vi "新记录通知.vi"() -> ()   [LabVIEW 2017]
uses:
  <vilib>/Utility/miscctls.llb/LVRowAndColumnTypeDef.ctl
  <vilib>/Utility/miscctls.llb/LVRowAndColumnUnsignedTypeDef.ctl
  <vilib>/Utility/inputDevices.llb/mouseAcquire.vi
panel:
  in  "列表菜单":enum16{"预览", "忽略此条", "删除缓存文件", "复制到剪贴板"}(ring)
  out "点到行列-实时列表":T1 caption="单元格位置"
  in  "device ID":refnum<k1> caption="设备ID"
  in  "新记录":cluster{"新记录列表行":string[], "对应缓存文件":string}[](array[cluster])
  in  "报警记录列表":i32[](listbox)
  in  "忽略全部":bool
  in  "预览全部":bool
  # "* 双击单元格打开预览\n  右键菜单中查看更多选项，管理界面中查看更多记录"
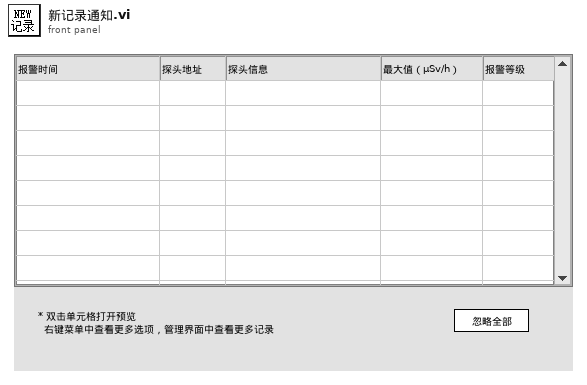
[diagram p1: front panel]
types:
  T1 = typedef "LVRowAndColumnTypeDef.ctl" = cluster{"Row":i32, "Column":i32}
  T2 = typedef "LVRowAndColumnUnsignedTypeDef.ctl" = cluster{"Row":u32, "Column":u32}
  T3 = enum32{"Invalid", "Standard", "Closed", "Hidden", "Minimized", "Maximized"}
  T4 = typedef "eventvkey.ctl" = enum16{"ASCII", "Enter", "Return", "Shift", "Ctrl", "Alt", "Cmd", "Opt", "Caps", "NumLock", "Clear", "Break", "Up", "Down", "Left", "Right", "Insert", "Delete", "Home", "End", "PageUp", "PageDown", "Escape", "Help", "Pause", "ScrollLock", "F1", "F2", "F3", "F4", "F5", "F6", "F7", "F8", "F9", "F10", "F11", "F12", "F13", "F14", "F15", "F16", "F17", "F18", "F19", "F20", "F21", "F22", "F23", "F24", "Play", "VolumeUp", "VolumeDown", "Mute", "Two Byte Char"}
  T5 = typedef "LVPoint32TypeDef.ctl" = cluster{"Horizontal":i32, "Vertical":i32}
  T6 = cluster{"button 1":bool, "button 2":bool, "button 3":bool, "button 4":bool}
  T7 = cluster{"Shift":bool, "Ctrl":bool, "Alt":bool, "Cmd":bool, "Opt":bool}
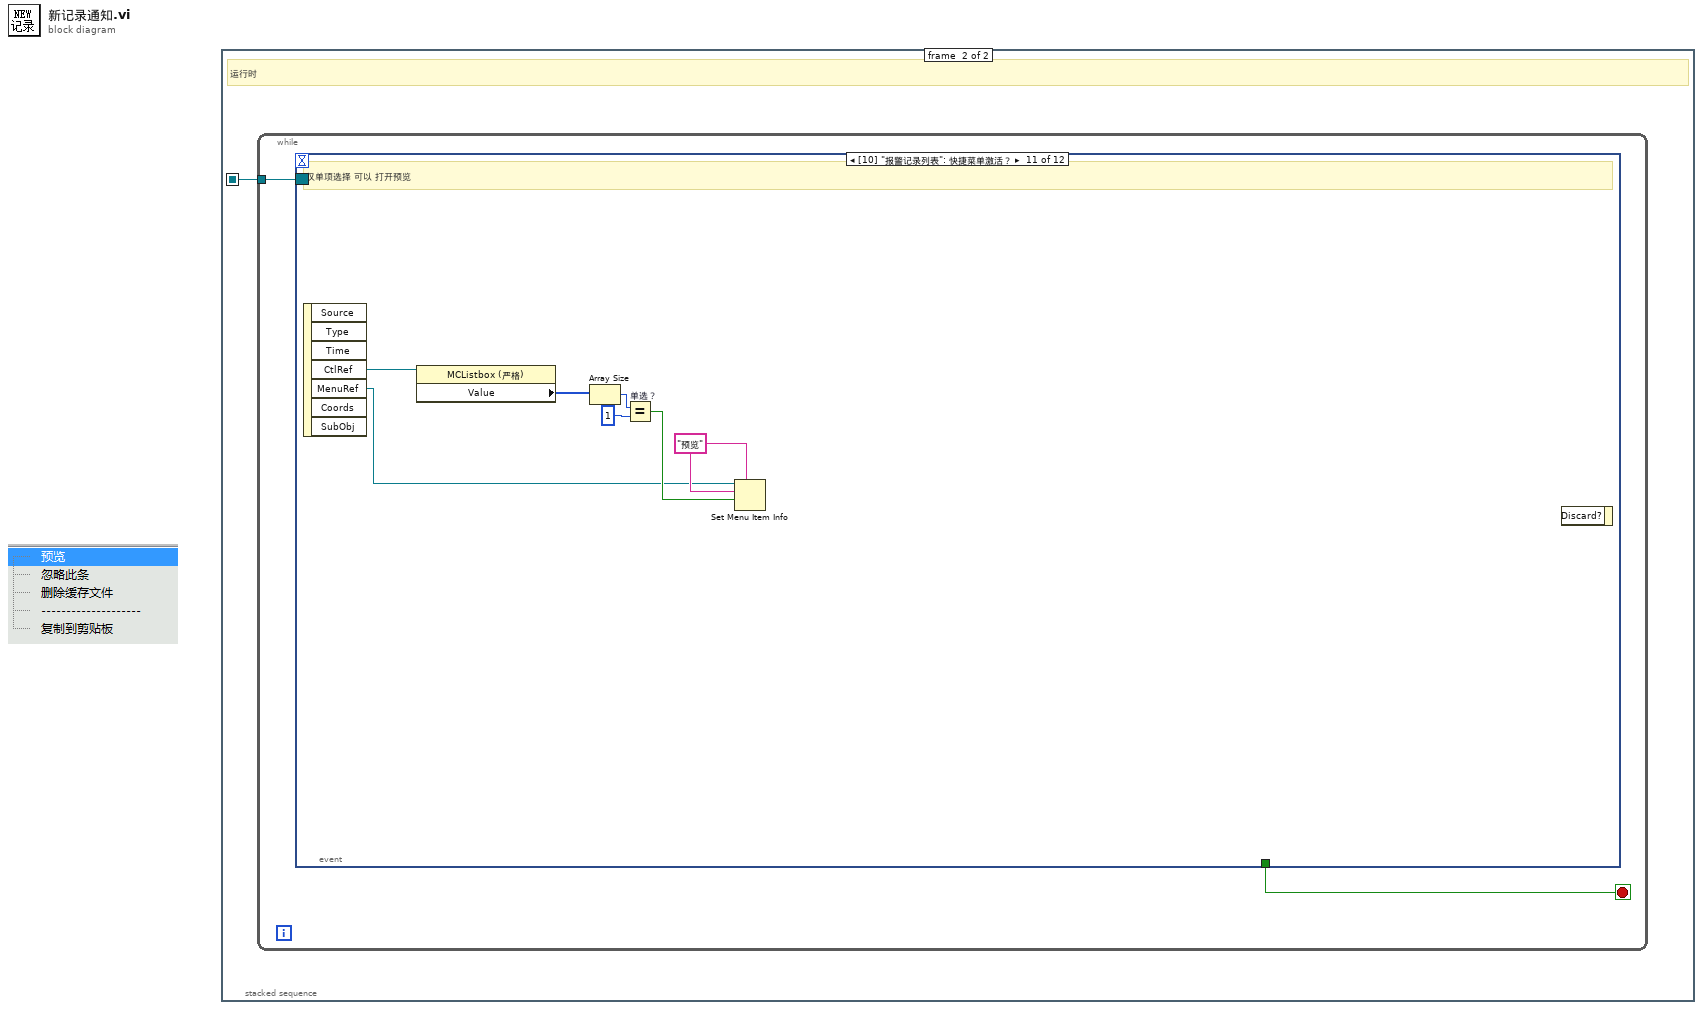
[diagram p0: block diagram]
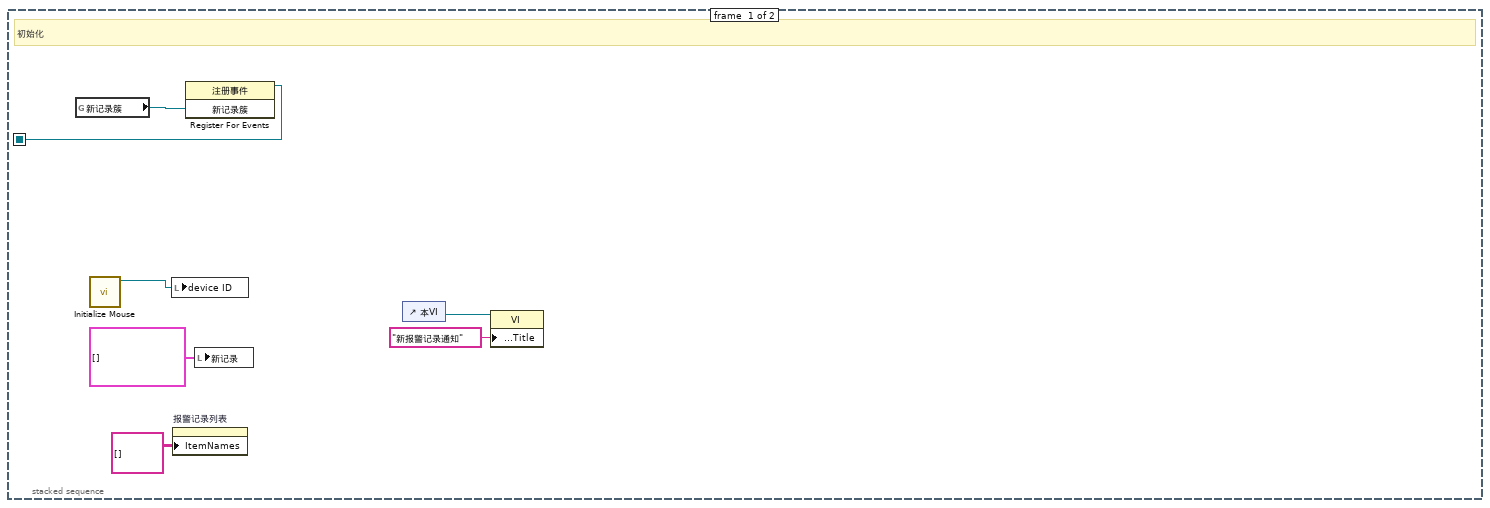
[diagram p2: hidden frame]
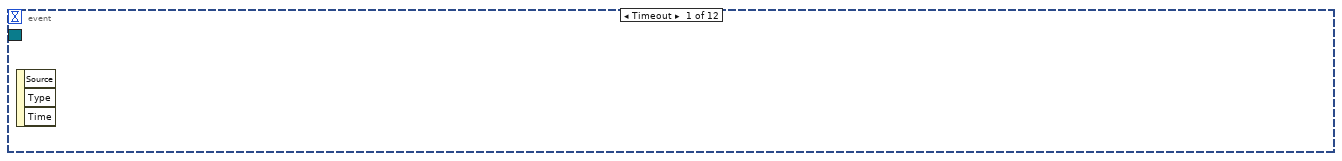
[diagram p3: hidden frame]
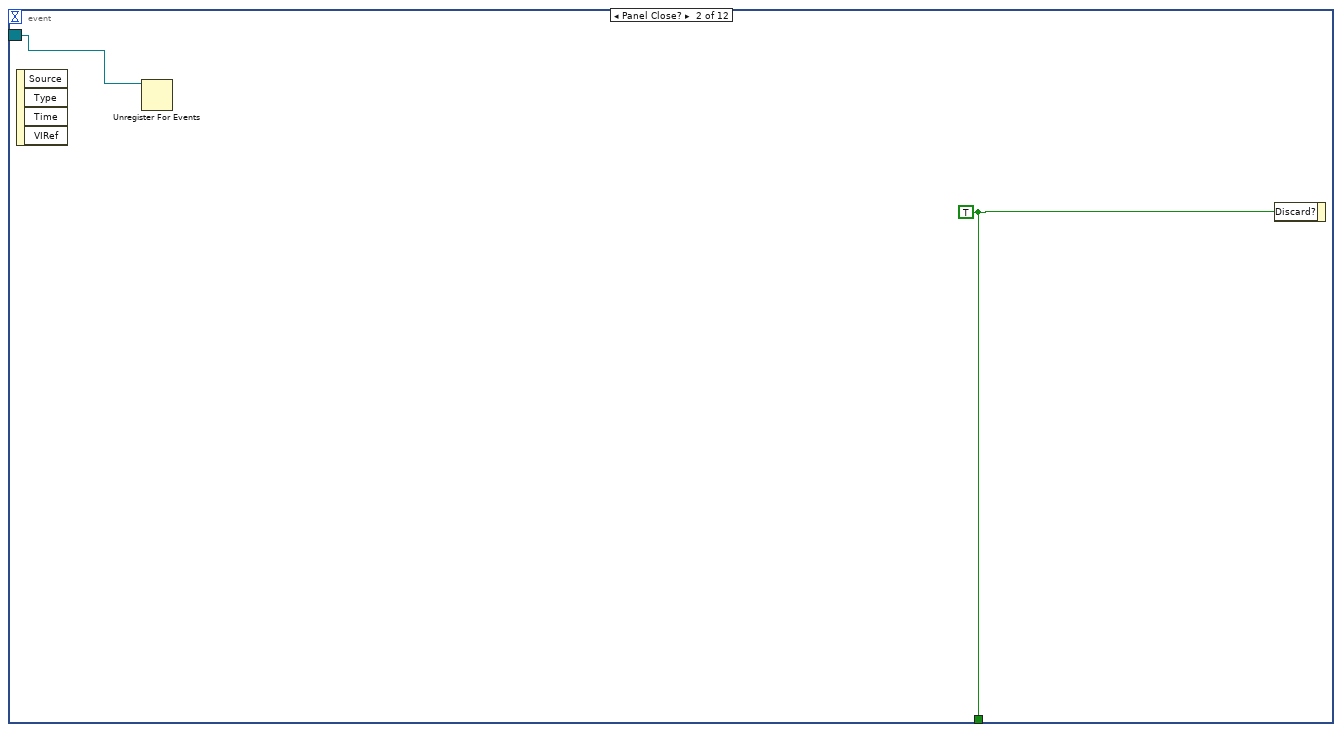
[diagram p4: hidden frame]
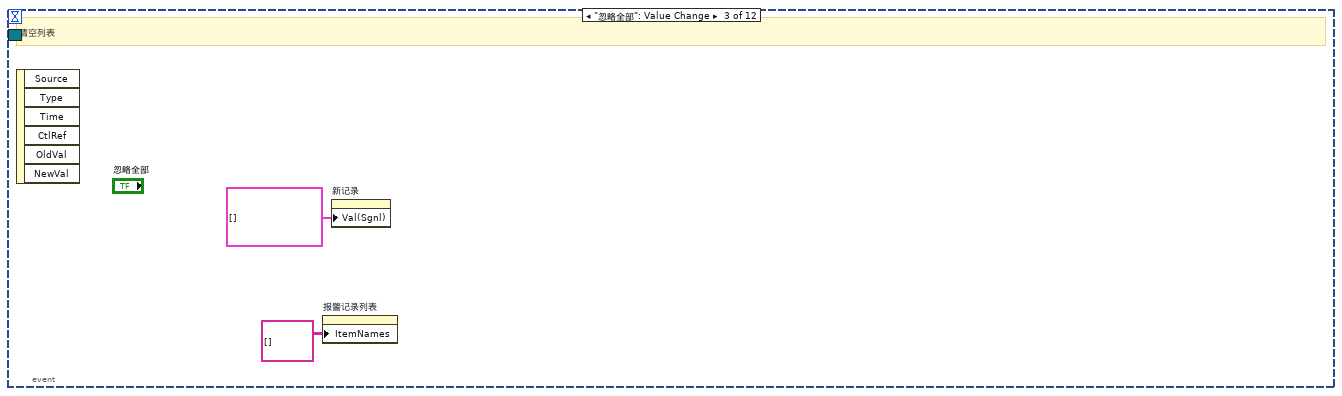
[diagram p5: hidden frame]
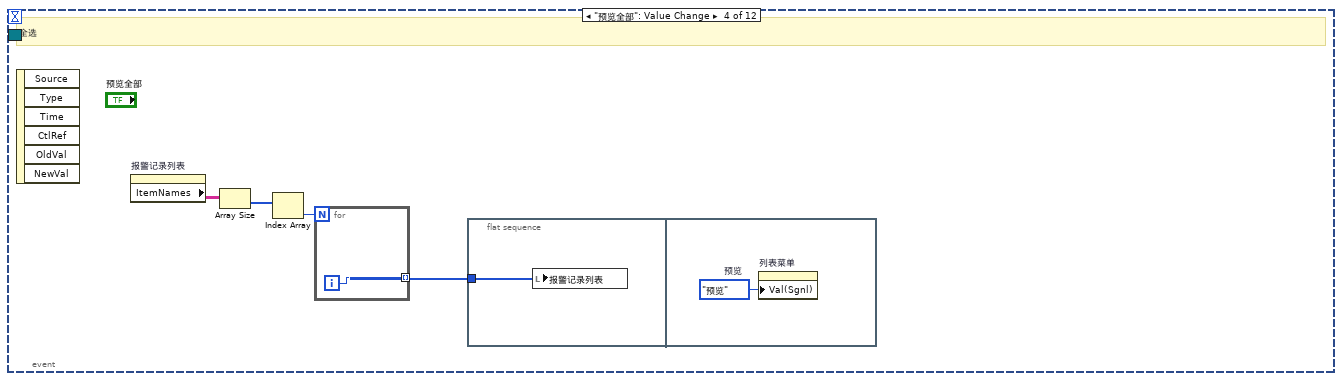
[diagram p6: hidden frame]
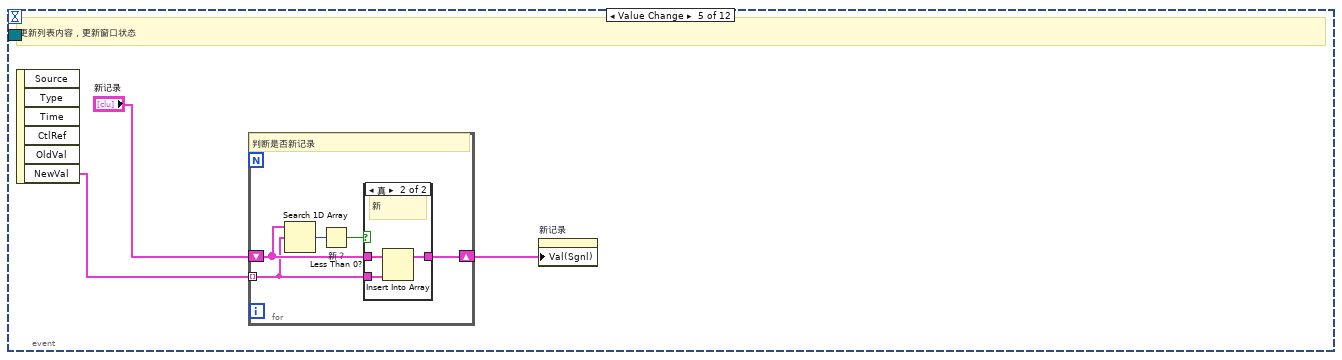
[diagram p7: hidden frame]
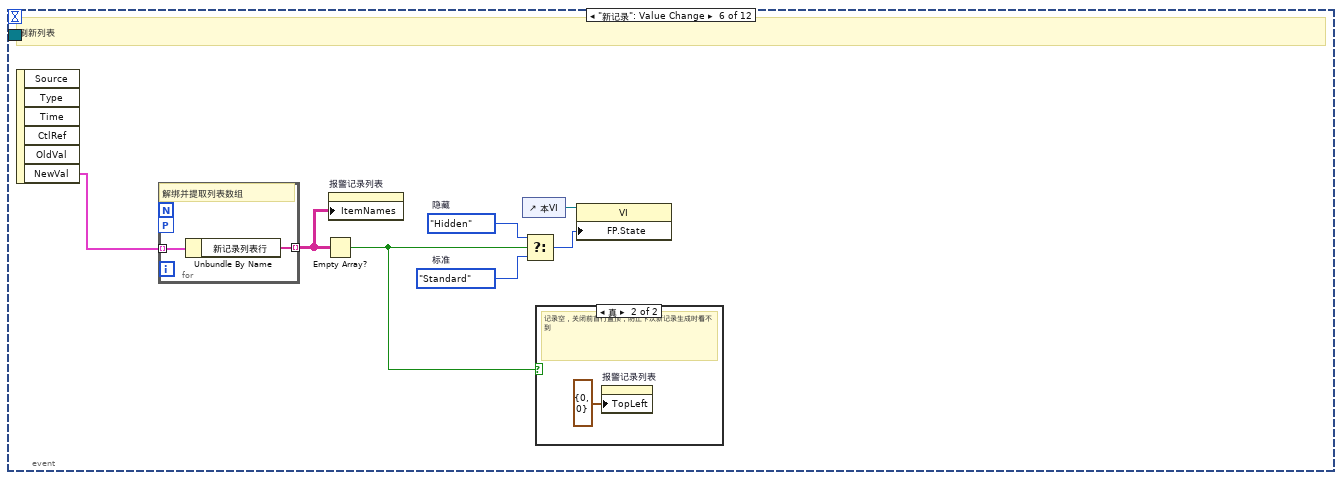
[diagram p9: hidden frame]
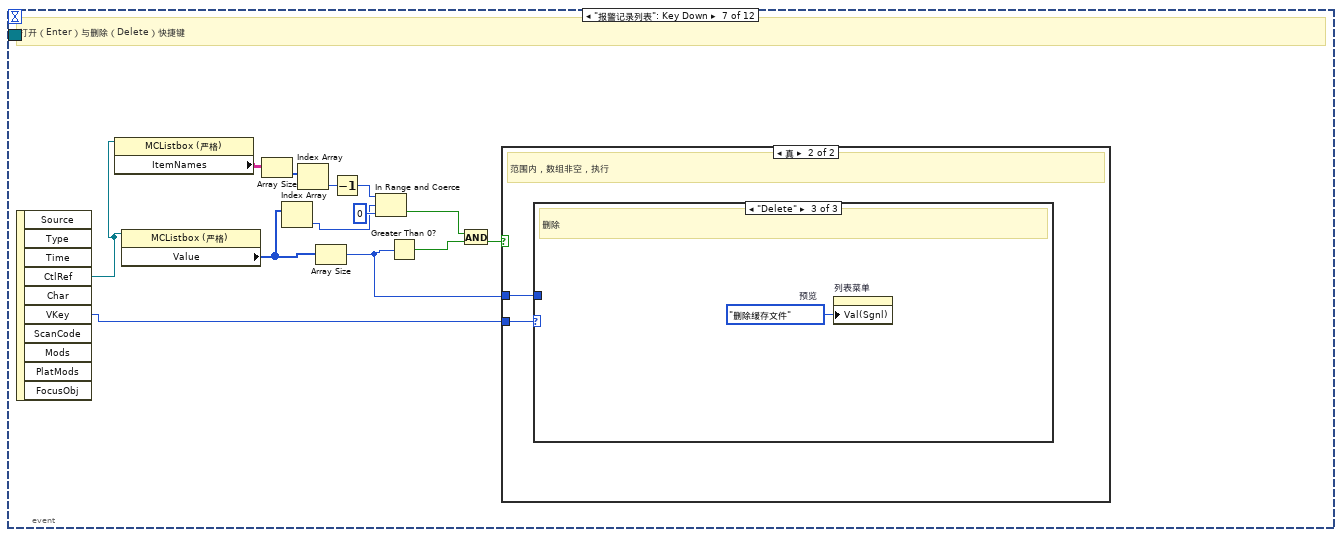
[diagram p11: hidden frame]
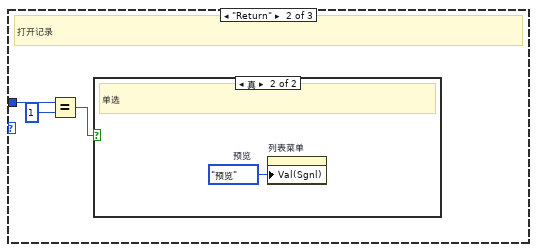
[diagram p14: hidden frame]
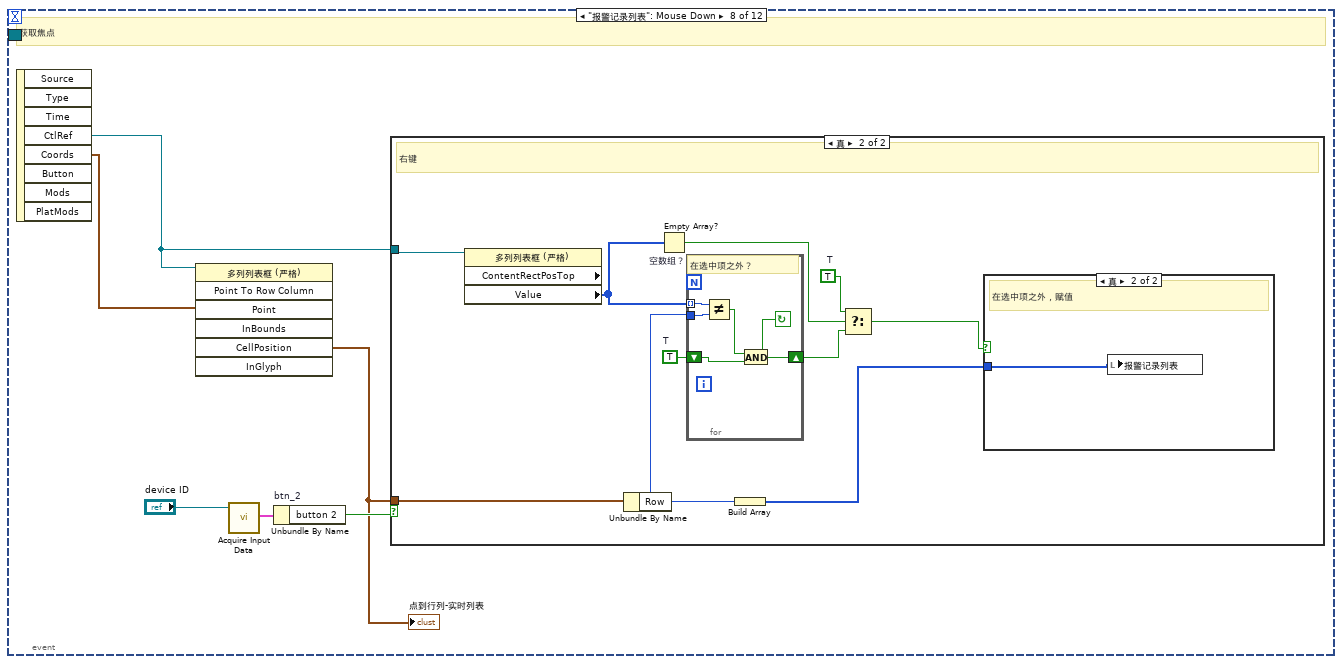
[diagram p16: hidden frame]
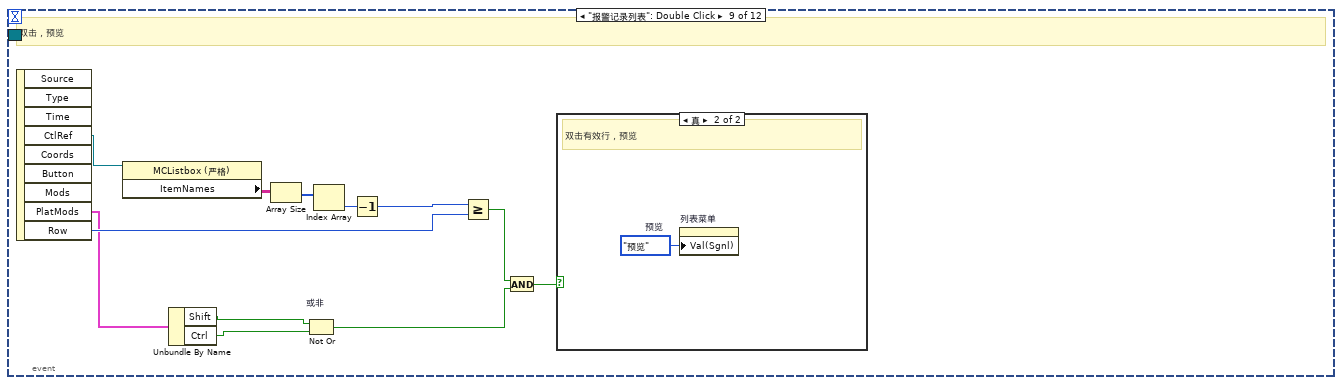
[diagram p19: hidden frame]
diagram:
  n1 = stacked-sequence {
    seq-local: [w6 _] -> [_ w8]
    frame #0 {
      # "初始化"
      n2 = global read "全局变量-35点监测.vi" "新记录簇"() -> (w7:refnum<vi>)
      n3 = call <vilib>:"Initialize Mouse.vi"() -> ("device ID"=w5:refnum<k1>)  [unwired: 10 in, 1 out]
      n4 = local write "device ID"(w5) -> ()
      n5 = property on="报警记录列表" class="MCListbox (严格)"("ItemNames"=string[][] [] ("项名")) -> ()  [unwired: 2 in, 2 out]
      n6 = register-events(w7) -> (reference out=w6:refnum<event-registration>)  [unwired: 2 in, 1 out]
      n7 = local write "新记录"(cluster{"新记录列表行":string[], "对应缓存文件":string}[] [] ("新记录")) -> ()
      n8 = control-ref of="本VI"() -> (w3:refnum<vi>)
      n9 = property class="VI"(reference=w3, "Front Panel.Title"="新报警记录通知" ("前面板窗口:标题")) -> ()  [unwired: 1 in, 2 out]
    }
    frame #1 {
      # "运行时"
      n10 = while {
        tunnel: w8 -> [w9]
        stop <- w10 stop-if-true
        n11 = event shown="[10] \"报警记录列表\": 快捷菜单激活？" {
          selector: w9 -> [_ w11 _ _ _ _ _ _ _ _ _ _]
          dyn-events: _ -> [_ _ _ _ _ _ _ _ _ _ _ _]
          timeout: _ -> [_ _ _ _ _ _ _ _ _ _ _ _]
          tunnel: [_ w12 _ _ _ _ _ _ _ _ _ _] -> w10
          event Timeout {
            n12 = event-data() -> ()  [unwired: 1 in, 3 out]
          }
          event Panel Close? {
            w12 = TRUE ("放弃？")
            n13 = event-data() -> ()  [unwired: 1 in, 4 out]
            n14 = Unregister For Events(event registration refnum=w11) -> ()  [unwired: 1 in, 1 out]
            n15 = event-data("Discard?"=w12) -> ()  [unwired: 1 in, 1 out]
          }
          event "忽略全部": Value Change {
            # "清空列表"
            n16 = event-data() -> ()  [unwired: 1 in, 6 out]
            n17 = property on="报警记录列表" class="MCListbox (严格)"("ItemNames"=string[][] [] ("项名")) -> ()  [unwired: 2 in, 2 out]
            n18 = property on="新记录" class="Arr (严格)"("Val(Sgnl)"=cluster{"新记录列表行":string[], "对应缓存文件":string}[] [] ("值(信号)")) -> ()  [unwired: 2 in, 2 out]
          }
          event "预览全部": Value Change {
            # "全选"
            n19 = event-data() -> ()  [unwired: 1 in, 6 out]
            n20 = property on="报警记录列表" class="MCListbox (严格)"() -> ("ItemNames"=w18:string[][])  [unwired: 2 in, 2 out]
            n21 = Array Size(array=w18) -> (size(s)=w17:i32[])
            n22 = Index Array(array=w17) -> (element=w16:i32)  [unwired: 1 in]
            n23 = for {
              N: w16 -> [_]
              tunnel: [w19] -> w15 mode=indexing
              i -> [w19]
            }
            n24 = flat-sequence {
              tunnel: w15 -> [w20]
              frame #0 {
                n25 = local write "报警记录列表"(w20) -> ()
              }
              frame #1 {
                w21 = enum16{"预览", "忽略此条", "删除缓存文件", "复制到剪贴板"}."预览"  # 预览
                n26 = property on="列表菜单" class="Enum (严格)"("Val(Sgnl)"=w21) -> ()  [unwired: 2 in, 2 out]
              }
            }
          }
          event Value Change {
            # "更新列表内容，更新窗口状态"
            n27 = event-data() -> ("NewVal"=w24:cluster{"新记录列表行":string[], "对应缓存文件":string}[])  [unwired: 1 in, 5 out]
            n28 = for {
              tunnel: w24 -> [w27] mode=indexing
              shift-right: [w29] -> w22
              shift-left: "新记录" -> [w28]
              # "判断是否新记录"
              n29 = Search 1D Array(1D array=w28, element=w27) -> (index of element=w26:i32)  [unwired: 1 in]
              n30 = Less Than 0? "新？"(x=w26) -> (x < 0?=w25:bool)
              n31 = case shown="真" w25 {
                tunnel: w28 -> [w30 w33]
                tunnel: w27 -> [_ w32]
                tunnel: [w30 w31] -> w29
                frame False {
                  # "非新"
                }
                frame True {
                  # "新"
                  n32 = Insert Into Array(array=w33, new element=w32) -> (w31:cluster{"新记录列表行":string[], "对应缓存文件":string}[])  [unwired: 1 in]
                }
              }
            }
            n33 = property on="新记录" class="Arr (严格)"("Val(Sgnl)"=w22) -> ()  [unwired: 2 in, 2 out]
          }
          event "新记录": Value Change {
            w38 = T3."Hidden"  # 隐藏
            w37 = T3."Standard"  # 标准
            # "刷新列表"
            n34 = event-data() -> ("NewVal"=w40:cluster{"新记录列表行":string[], "对应缓存文件":string}[])  [unwired: 1 in, 5 out]
            n35 = for {
              workers-P: _ -> [_]
              tunnel: w40 -> [w43] mode=indexing
              tunnel: [w42] -> w35 mode=indexing
              # "解绑并提取列表数组"
              n36 = Unbundle By Name(w43) -> ("新记录列表行"=w42:string[])
            }
            n37 = Empty Array?(array=w35) -> (empty?=w34:bool)
            n38 = property on="报警记录列表" class="MCListbox (严格)"("ItemNames"=w35) -> ()  [unwired: 2 in, 2 out]
            n39 = control-ref of="本VI"() -> (w39:refnum<vi>)
            n40 = Select(t=w38, s=w34, f=w37) -> (s? t:f=w36:T3)
            n41 = case shown="真" w34 {
              frame False {
              }
              frame True {
                # "记录空，关闭前首行置顶，防止下次新记录生成时看不到"
                n42 = property on="报警记录列表" class="MCListbox (严格)"("TopLeft"=T2 {"Row"=0, "Column"=0} ("左上可见单元格")) -> ()  [unwired: 2 in, 2 out]
              }
            }
            n43 = property class="VI"(reference=w39, "FP.State"=w36) -> ()  [unwired: 1 in, 2 out]
          }
          event "报警记录列表": Key Down {
            # "打开（Enter）与删除（Delete）快捷键"
            n44 = event-data() -> ("CtlRef"=w49:refnum<vi>, "VKey"=w54:T4)  [unwired: 1 in, 8 out]
            n45 = property class="MCListbox (严格)"(reference=w49) -> ("ItemNames"=w50:string[][])  [unwired: 1 in, 2 out]
            n46 = property class="MCListbox (严格)"(reference=w49) -> ("Value"=w47:i32[])  [unwired: 1 in, 2 out]
            n47 = Array Size(array=w50) -> (size(s)=w51:i32[])
            n48 = Index Array(array=w47) -> (element=w46:i32)  [unwired: 1 in]
            n49 = Index Array(array=w51) -> (element=w52:i32)  [unwired: 1 in]
            n50 = Array Size(array=w47) -> (size(s)=w55:i32)
            n51 = Decrement(x=w52) -> (x-1=w53:i32)
            n52 = In Range and Coerce(upper limit=w53, x=w46, lower limit=0 ("下限")) -> (In Range?=w44:bool)  [unwired: 1 out]
            n53 = Greater Than 0?(x=w55) -> (x > 0?=w56:bool)
            n54 = And(x=w44, y=w56) -> (x .and. y?=w45:bool)
            n55 = case shown="真" w45 {
              tunnel: w55 -> [_ w58]
              tunnel: w54 -> [_ w57]
              frame False {
                # "数组空，不执行"
              }
              frame True {
                # "范围内，数组非空，执行"
                n56 = case shown="\"Delete\"" w57 {
                  tunnel: w58 -> [_ w61 _]
                  frame "ASCII", Default {
                    # "不执行"
                  }
                  frame "Return" {
                    # "打开记录"
                    n57 = Equal?(x=w61, y=1) -> (x = y?=w59:bool)
                    n58 = case shown="真" w59 {
                      frame False {
                        # "多选"
                      }
                      frame True {
                        w62 = enum16{"预览", "忽略此条", "删除缓存文件", "复制到剪贴板"}."预览"  # 预览
                        # "单选"
                        n59 = property on="列表菜单" class="Enum (严格)"("Val(Sgnl)"=w62) -> ()  [unwired: 2 in, 2 out]
                      }
                    }
                  }
                  frame "Delete" {
                    w63 = enum16{"预览", "忽略此条", "删除缓存文件", "复制到剪贴板"}."删除缓存文件"  # 预览
                    # "删除"
                    n60 = property on="列表菜单" class="Enum (严格)"("Val(Sgnl)"=w63) -> ()  [unwired: 2 in, 2 out]
                  }
                }
              }
            }
          }
          event "报警记录列表": Mouse Down {
            # "获取焦点"
            n61 = event-data() -> ("CtlRef"=w65:refnum<vi>, "Coords"=w66:T5)  [unwired: 1 in, 6 out]
            n62 = invoke class="多列列表框 (严格)" method="Point To Row Column"(reference=w65, "Point"=w66) -> ("CellPosition"=w64:T1)  [unwired: 5 in, 6 out]
            "点到行列-实时列表" <- w64
            n63 = call-poly <vilib>:"Acquire Input Data.vi"("device ID"="device ID") -> ("button info"=w68:T6)  [unwired: 15 in, 3 out]
            n64 = Unbundle By Name "btn_2"(w68) -> ("button 2"=w69:bool)
            n65 = case shown="真" w69 {
              tunnel: w65 -> [_ w78]
              tunnel: w64 -> [_ w75]
              frame False {
                # "不是右键"
              }
              frame True {
                w72 = TRUE  # T
                w79 = TRUE  # T
                # "右键"
                n66 = property class="多列列表框 (严格)" props=["ContentRectPosTop", "Value"](reference=w78) -> ("Value"=w74:i32[])  [unwired: 1 in, 3 out]
                n67 = Unbundle By Name(w75) -> ("Row"=w77:i32)
                n68 = Empty Array? "空数组？"(array=w74) -> (empty?=w73:bool)
                n69 = for {
                  tunnel: w74 -> [w85] mode=indexing
                  shift-right: [w82] -> w71
                  shift-left: w79 -> [w83]
                  tunnel: w77 -> [w81]
                  stop <- w82 continue-if-true
                  # "在选中项之外？"
                  n70 = Not Equal?(x=w85, y=w81) -> (x != y?=w84:bool)
                  n71 = And(x=w84, y=w83) -> (x .and. y?=w82:bool)
                }
                n72 = Build Array(w77) -> (w76:i32[])
                n73 = Select(t=w72, s=w73, f=w71) -> (s? t:f=w70:bool)
                n74 = case shown="真" w70 {
                  tunnel: w76 -> [_ w80]
                  frame False {
                    # "在选中项之中，不赋值"
                  }
                  frame True {
                    # "在选中项之外，赋值"
                    n75 = local write "报警记录列表"(w80) -> ()
                  }
                }
              }
            }
          }
          event "报警记录列表": Double Click {
            # "双击，预览"
            n76 = event-data() -> ("CtlRef"=w87:refnum<vi>, "PlatMods"=w91:T7, "Row"=w94:i32)  [unwired: 1 in, 6 out]
            n77 = property class="MCListbox (严格)"(reference=w87) -> ("ItemNames"=w97:string[][])  [unwired: 1 in, 2 out]
            n78 = Unbundle By Name(w91) -> ("Shift"=w90:bool, "Ctrl"=w89:bool)
            n79 = Array Size(array=w97) -> (size(s)=w96:i32[])
            n80 = Not Or "或非"(1:w89, 2:w90) -> (0:w92:bool)
            n81 = Index Array(array=w96) -> (element=w95:i32)  [unwired: 1 in]
            n82 = Decrement(x=w95) -> (x-1=w86:i32)
            n83 = Greater Or Equal?(x=w86, y=w94) -> (x >= y?=w93:bool)
            n84 = And(x=w93, y=w92) -> (x .and. y?=w88:bool)
            n85 = case shown="真" w88 {
              frame False {
                # "无效行"
              }
              frame True {
                w98 = enum16{"预览", "忽略此条", "删除缓存文件", "复制到剪贴板"}."预览"  # 预览
                # "双击有效行，预览"
                n86 = property on="列表菜单" class="Enum (严格)"("Val(Sgnl)"=w98) -> ()  [unwired: 2 in, 2 out]
              }
            }
          }
          event "报警记录列表": Shortcut Menu Selection (User) {
            # "触发菜单事件"
            n87 = event-data() -> ("ItemTag"=w100:string)  [unwired: 1 in, 7 out]
            n88 = property on="列表菜单" class="Enum (严格)"() -> ("Strings []"=w101:string[])  [unwired: 2 in, 2 out]
            n89 = for {
              tunnel: w101 -> [w105] mode=indexing
              tunnel: w100 -> [w104]
              tunnel: [w102] -> w99
              i -> [w102]
              stop <- w103 stop-if-true
              # "寻找匹配项"
              n90 = Equal?(x=w105, y=w104) -> (x = y?=w103:bool)
            }
            n91 = property on="列表菜单" class="Enum (严格)"("Val(Sgnl)"=w99) -> ()  [unwired: 2 in, 2 out]
          }
          event "报警记录列表": Shortcut Menu Activation? {
            w110 = "预览" ("项标识符")
            # "仅单项选择 可以 打开预览"
            n92 = event-data() -> ("CtlRef"=w112:refnum<vi>, "MenuRef"=w106:refnum<k9>)  [unwired: 1 in, 5 out]
            n93 = property class="MCListbox (严格)"(reference=w112) -> ("Value"=w107:i32[])  [unwired: 1 in, 2 out]
            n94 = Array Size(array=w107) -> (size(s)=w108:i32)
            n95 = Equal? "单选？"(x=w108, y=1) -> (x = y?=w111:bool)
            n96 = Set Menu Item Info(7:w110, 9:w111, 10:w110, 11:w106) -> ()  [unwired: 3 in, 2 out]
            n97 = event-data() -> ()  [unwired: 2 in, 1 out]
          }
          event "列表菜单": Value Change {
            # "菜单事件"
            n98 = event-data() -> ("NewVal"=w115:enum16{"预览", "忽略此条", "删除缓存文件", "复制到剪贴板"})  [unwired: 1 in, 5 out]
            n99 = local read "新记录"() -> (w113:cluster{"新记录列表行":string[], "对应缓存文件":string}[])
            n100 = case shown="\"预览\", 默认" w115 {
              tunnel: "报警记录列表" -> [w125 w149 w154 w178]
              tunnel: w113 -> [w124 w147 w155 _]
              frame "预览", Default {
                # "打开预览窗口"
                n101 = call "路径查找创建-报警记录清单.vi"() -> ("缓存数据文件夹"=w123:path)  [unwired: 8 in, 11 out]
                n102 = Index Array(array=w125) -> (element=w119:i32)  [unwired: 1 in]
                n103 = Index Array(array=w124, index=w119) -> (element=w122:cluster{"新记录列表行":string[], "对应缓存文件":string})
                n104 = Unbundle By Name(w122) -> ("对应缓存文件"=w121:string)
                n105 = Build Path(base path=w123, name or relative path=w121) -> (appended path=w120:path)
                n106 = vi-ref "生成报表.vi"() -> (w116:refnum<vi>)
                n107 = call <vilib>:"Check if File or Folder Exists.vi"("path"=w120) -> ("file or folder exists?"=w118:bool, "dup path"=w117:path)  [unwired: 8 in, 1 out]
                n108 = case shown="真" w118 {
                  tunnel: w117 -> [_ w129]
                  tunnel: w116 -> [_ w128]
                  frame False {
                    n109 = call "显示对话框信息2"() -> ("忽略此条"=w126:bool)  [unwired: 10 in, 1 out]
                    n110 = stacked-sequence {
                      tunnel: w126 -> [_]
                      frame #0 {
                        n111 = property on="列表菜单" class="Enum (严格)"("Val(Sgnl)"=enum16{"预览", "忽略此条", "删除缓存文件", "复制到剪贴板"}."忽略此条" ("值(信号)")) -> ()  [unwired: 2 in, 2 out]
                      }
                    }
                  }
                  frame True {
                    # "有效文件"
                    n112 = invoke class="VI" method="FP.Open"(reference=w128, "Activate"=TRUE ("激活？"), "State"=T3."Hidden" ("状态")) -> (reference out=w132:refnum<vi>, error out=w144:errorcluster)  [unwired: 2 in, 3 out]
                    n113 = call "通过控件名获取控件引用.vi"("控件名数组"=string[] ["缓存数据路径"], "VI引用"=w132) -> ("控件引用输出"=w134:refnum<vi>[], "VI引用o"=w136:refnum<vi>)  [unwired: 7 in, 1 out]
                    n114 = Index Array(array=w134) -> (element=w135:refnum<vi>)  [unwired: 1 in]
                    n115 = property class="Ctl"(reference=w135, error in=w144, "Val(Sgnl)"=w129) -> (error out=w145:errorcluster)  [unwired: 1 out]
                    n116 = invoke class="VI" method="Run VI"(reference=w136, error in=w145, "Wait until done"=FALSE ("结束前等待"), "Auto Dispose Ref"=TRUE ("自动销毁引用")) -> (reference out=w139:refnum<vi>, error out=w140:errorcluster)  [unwired: 1 in, 3 out]
                    n117 = invoke class="VI" method="FP.Open"(reference=w139, error in=w140, "Activate"=TRUE ("激活？"), "State"=T3."Standard" ("状态")) -> (error out=w143:errorcluster)  [unwired: 1 in, 4 out]
                    n118 = call <vilib>:"Clear Errors.vi"("error in (no error)"=w143) -> ()  [unwired: 5 in, 2 out]
                  }
                }
              }
              frame "忽略此条" {
                # "从“新记录”中删除，不删除缓存文件"
                n119 = Reverse 1D Array(array=w149) -> (reversed array=w148:i32[])
                n120 = for {
                  tunnel: w148 -> [w150] mode=indexing
                  shift-right: [w151] -> w146
                  shift-left: w147 -> [w152]
                  # "删除忽略项"
                  n121 = Delete From Array(array=w152, index=w150) -> (array with subset deleted=w151:cluster{"新记录列表行":string[], "对应缓存文件":string}[])  [unwired: 1 in, 1 out]
                }
                n122 = property on="新记录" class="Arr (严格)"("Val(Sgnl)"=w146) -> ()  [unwired: 2 in, 2 out]
              }
              frame "删除缓存文件" {
                # "删除缓存文件，刷新列表"
                n123 = call "显示对话框信息"() -> ("确定"=w153:bool)  [unwired: 10 in, 1 out]
                n124 = case shown="真" w153 {
                  tunnel: w155 -> [_ w157]
                  tunnel: w154 -> [_ w156]
                  frame False {
                    # "取消删除"
                  }
                  frame True {
                    # "确认删除"
                    n125 = stacked-sequence {
                      tunnel: w157 -> [w162 _]
                      tunnel: w156 -> [w161 _]
                      frame #0 {
                        # "删除文件，刷新列表"
                        n126 = call "路径查找创建-报警记录清单.vi"() -> ("缓存数据文件夹"=w158:path)  [unwired: 8 in, 11 out]
                        n127 = Reverse 1D Array(array=w161) -> (reversed array=w160:i32[])
                        n128 = for {
                          tunnel: w160 -> [w169] mode=indexing
                          shift-right: [w164] -> w159
                          shift-left: w162 -> [w170]
                          tunnel: w158 -> [w163]
                          # "删除文件与列表项"
                          n129 = Delete From Array(array=w170, index=w169) -> (deleted portion=w168:cluster{"新记录列表行":string[], "对应缓存文件":string}, array with subset deleted=w164:cluster{"新记录列表行":string[], "对应缓存文件":string}[])  [unwired: 1 in]
                          n130 = Unbundle By Name(w168) -> ("对应缓存文件"=w167:string)
                          n131 = Build Path(base path=w163, name or relative path=w167) -> (appended path=w165:path)
                          n132 = Delete(path (use dialog)=w165) -> (error out=w166:errorcluster)  [unwired: 4 in, 2 out]
                          n133 = call <vilib>:"Clear Errors.vi"("error in (no error)"=w166) -> ()  [unwired: 5 in, 2 out]
                        }
                        n134 = property on="新记录" class="Arr (严格)"("Val(Sgnl)"=w159) -> ()  [unwired: 2 in, 2 out]
                      }
                      frame #1 {
                        w171 = enum16{"刷新", "预览并生成报表", "删除记录", "复制选中项至剪贴板"}."刷新"  # 刷新
                        # "通知“管理VI”刷新报警记录列表"
                        n135 = vi-ref "多点监测上位机.vi"() -> (w175:refnum<vi>)
                        n136 = call "通过控件名获取控件引用.vi"("控件名数组"=string[] ["菜单项-报警列表"], "VI引用"=w175) -> ("控件引用输出"=w173:refnum<vi>[])  [unwired: 7 in, 2 out]
                        n137 = Index Array(array=w173) -> (element=w172:refnum<vi>)  [unwired: 1 in]
                        n138 = property class="Ctl"(reference=w172, "Val(Sgnl)"=w171) -> ()  [unwired: 1 in, 2 out]
                      }
                    }
                  }
                }
              }
              frame "复制到剪贴板" {
                # "筛选选中项，到剪贴板"
                n139 = property on="报警记录列表" class="MCListbox (严格)"() -> ("ItemNames"=w179:string[][])  [unwired: 2 in, 2 out]
                n140 = for {
                  tunnel: w179 -> [w191]
                  tunnel: w178 -> [w189] mode=indexing
                  shift-right: [w187] -> w176
                  shift-left: string[][] [] ("ItemNames") -> [w190]
                  # "筛选选中项"
                  n141 = Index Array(array=w191, index (row)=w189) -> (element=w188:string[])  [unwired: 1 in]
                  n142 = Insert Into Array(array=w190, new element=w188) -> (w187:string[][])  [unwired: 2 in]
                }
                n143 = Array To Spreadsheet String(array=w176, 3:"%s" ("格式字符串")) -> (spreadsheet string=w184:string)  [unwired: 1 in]
                n144 = Array To Spreadsheet String(array=string[] ["报警时间", "探头编号", "探头信息", "最大值（μSv/h）", "报警等级"] ("ItemNames"), 3:"%s" ("格式字符串")) -> (spreadsheet string=w186:string)  [unwired: 1 in]
                n145 = control-ref of="本应用程序"() -> (w181:refnum<vi>)
                n146 = Concatenate Strings(w186, w184) -> (w185:string)
                n147 = invoke class="App" method="Clipboard.Write"(reference=w181, "Param 0"=w185) -> ()  [unwired: 2 in, 4 out]
              }
            }
          }
        }
      }
    }
  }
